vi "Collect information from UI to run measurement.vi"(8 "error in (no error)":errorcluster, 11 "Measurement UI in":refnum<class "Measurement UI.lvclass">) -> (0 "error out":errorcluster, 1 "Show UI?":bool, 2 "Device Names":string[](array[string]), 3 "Measurement UI out":refnum<class "Measurement UI.lvclass">, 4 "String":string, 5 "Measurement Name":string)   [LabVIEW 2015, in "Measurement UI.lvlib" / "Measurement UI.lvclass"]
uses:
  Measurement UI.lvclass
  Measurement UI.lvclass/Measurement UI.ctl
  Accessors/Read Measurement.vi
  Accessors/Read Power Supply.vi
  Accessors/Read Digitizer.vi
  Accessors/Read Function Generator.vi
  Read Multimeter.vi
  Accessors/Read Show FP_.vi
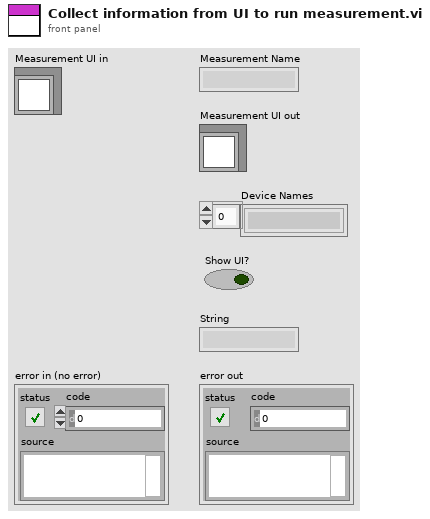
[diagram p1: front panel]
types:
  T1 = enum8{"Enabled", "Disabled", "Disabled and Grayed Out"}
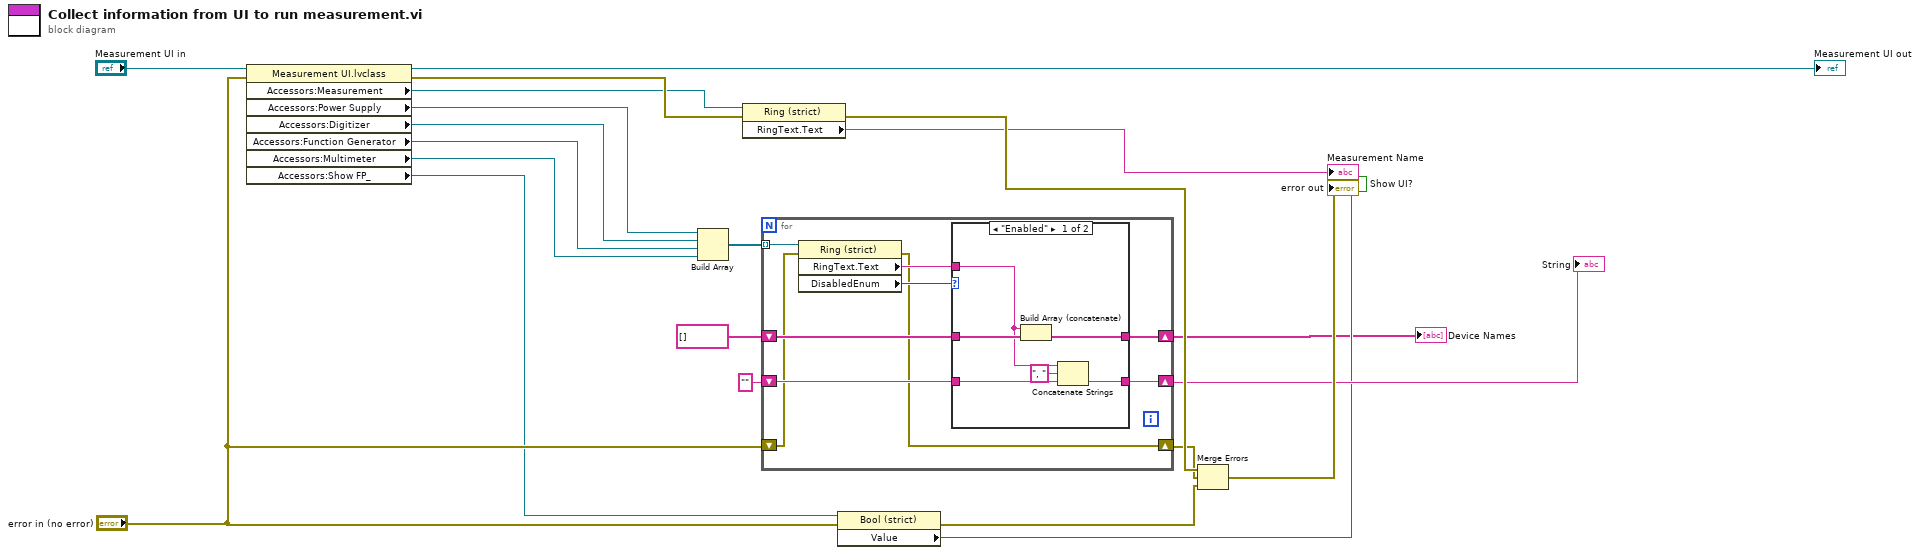
[diagram p0: block diagram]
diagram:
  n1 = property class="Measurement UI.lvclass"(reference="Measurement UI in", error in="error in (no error)") -> (reference out=→"Measurement UI out":refnum<class "Measurement UI.lvclass">, error out=w16:errorcluster, "Accessors:Measurement"=w15:refnum<vi>, "Accessors:Power Supply"=w14:refnum<vi>, "Accessors:Digitizer"=w13:refnum<vi>, "Accessors:Function Generator"=w12:refnum<vi>, "Accessors:Multimeter"=w11:refnum<vi>, "Accessors:Show FP_"=w10:refnum<vi>)
  n2 = Build Array(w14, w13, w12, w11) -> (w3:refnum<vi>[])
  n3 = property class="Ring (strict)"(reference=w15, error in=w16) -> (error out=w20:errorcluster, "RingText.Text"=→"Measurement Name":string)  [unwired: 1 out]
  n4 = for {
    shift-right: [w27] -> w2
    shift-left: string[] [] ("Device Names") -> [w26]
    tunnel: w3 -> [w30] mode=indexing
    shift-right: [w25] -> w7
    shift-left: "" -> [w24]
    shift-right: [w23] -> w18
    shift-left: "error in (no error)" -> [w22]
    n5 = property class="Ring (strict)"(reference=w30, error in=w22) -> (error out=w23:errorcluster, "RingText.Text"=w28:string, "DisabledEnum"=w29:T1)  [unwired: 1 out]
    n6 = case shown="\"Enabled\"" w29 {
      tunnel: w28 -> [w32 _]
      tunnel: [w36 w38] -> w27
      tunnel: w26 -> [w35 w38]
      tunnel: [w34 w37] -> w25
      tunnel: w24 -> [w33 w37]
      frame "Enabled" {
        n7 = Build Array (concatenate)(w32, w35) -> (w36:string[])
        n8 = Concatenate Strings(w32, ", " ("string"), w33) -> (w34:string)
      }
      frame "Disabled", Default {
      }
    }
  }
  "String" <- w7
  "Device Names" <- w2
  n9 = property class="Bool (strict)"(reference=w10, error in="error in (no error)") -> (error out=w19:errorcluster, "Value"=→"Show UI?":bool)  [unwired: 1 out]
  n10 = Merge Errors(w20, w18, w19) -> (→"error out":errorcluster)
